vi "Update Analysis Graph.vi"(8 "error in (no error)":errorcluster, 9 "Image Series":u16[][][](array[numeric]), 10 "Analysis Image":dbl[][](array[numeric]), 11 "Analysis Graph in":refnum<class "Analysis Graph.lvclass">) -> (0 "error out":errorcluster, 1 "Image Series  out":u16[][][](array[numeric]), 2 "Cursor.Cursor Position":T1, 3 "Analysis Graph out":refnum<class "Analysis Graph.lvclass">)   [LabVIEW 2023, in "Analysis Graph.lvclass"]
uses:
  Analysis Graph.lvclass
  Analysis Graph.lvclass/Analysis Graph.ctl
  Detail Graph/Detail Graph.lvclass
  Series Graph/Series Graph.lvclass
  <vilib>/Utility/miscctls.llb/LVPointDoubleTypeDef.ctl
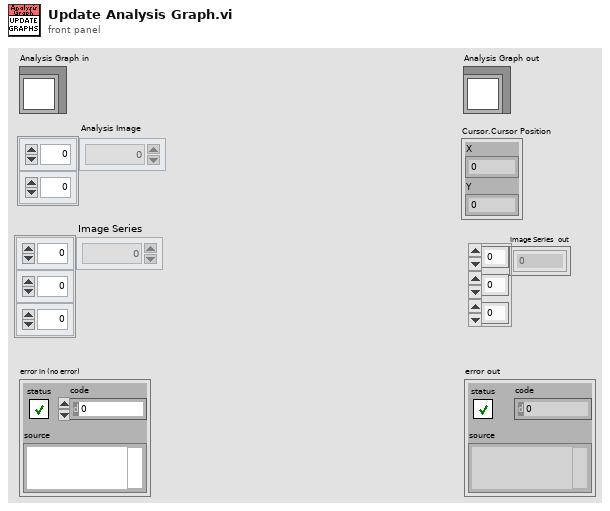
[diagram p1: front panel]
types:
  T1 = typedef "LVPointDoubleTypeDef.ctl" = cluster{"X":dbl, "Y":dbl}
  T2 = cluster{"ROI X":cluster{"Index":u32, "Length":u32}, "ROI Y":cluster{"Index":u32, "Length":u32}, "ROI Z":cluster{"Index":u32, "Length":u32}}
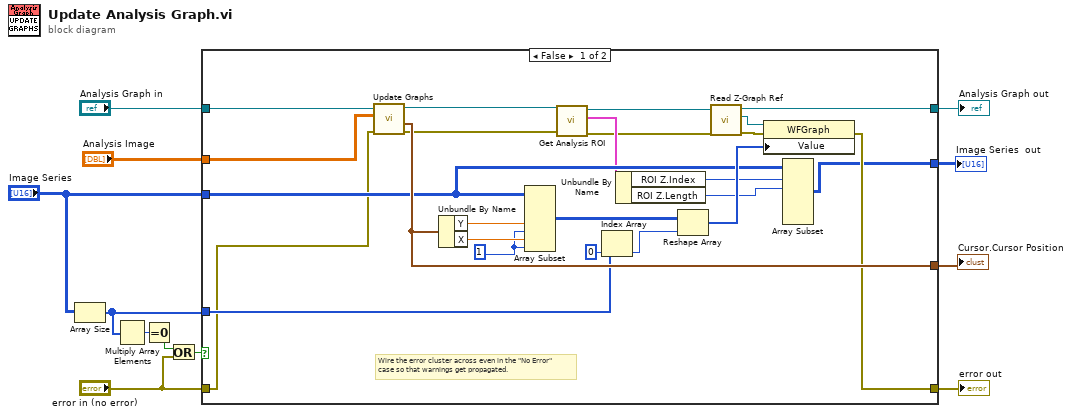
[diagram p0: block diagram]
diagram:
  n1 = Array Size(array="Image Series") -> (size(s)=w5:i32[])
  n2 = Multiply Array Elements(1:w5) -> (0:w9:i32)
  n3 = Equal To 0?(x=w9) -> (x = 0?=w8:bool)
  n4 = Or(x=w8, y="error in (no error)") -> (x .or. y?=w7:bool)
  n5 = case shown="False" w7 {
    tunnel: [w28 w39] -> w12
    tunnel: [w33 w40] -> w10
    tunnel: "Analysis Graph in" -> [w18 w40]
    tunnel: "error in (no error)" -> [w17 w39]
    tunnel: w5 -> [w23 _]
    tunnel: "Analysis Image" -> [w30 _]
    tunnel: "Image Series" -> [w26 w38]
    tunnel: [w29 _] -> w2
    tunnel: [w27 w38] -> w1
    frame False {
      w35 = 1 ("length")
      # "Wire the error cluster across even in the \"No Error\"\ncase so that warnings get propagated."
      n6 = call "Update Graphs.vi"("error in (no error)"=w17, "image"=w30, "Detail Graph in"=w18) -> ("error out"=w20:errorcluster, "Cursor.Cursor Position"=w29:T1, "Detail Graph out"=w14:refnum<class "Analysis Graph.lvclass">)  [unwired: 6 in]
      n7 = Unbundle By Name(w29) -> ("Y"=w37:dbl, "X"=w36:dbl)
      n8 = Array Subset(array=w26, index (dim 1)=w37, length (dim 1)=w35, index (dim 2)=w36, length (dim 2)=w35) -> (w22:u16[][][])  [unwired: 2 in]
      n9 = call "Get Analysis ROI.vi"("error in (no error)"=w20, "Analysis Graph in"=w14) -> ("error out"=w19:errorcluster, "ROI XYZ"=w21:T2, "Analysis Graph out"=w13:refnum<class "Analysis Graph.lvclass">)  [unwired: 7 in]
      n10 = Index Array(array=w23, index=0) -> (element=w25:i32)
      n11 = Unbundle By Name(w21) -> ("ROI Z.Index"=w16:u32, "ROI Z.Length"=w15:u32)
      n12 = Reshape Array(w22, w25) -> (w34:u16[])
      n13 = call "Read Z-Graph Ref.vi"("error in (no error)"=w19, "Series Graph in"=w13) -> ("error out"=w31:errorcluster, "Z-Graph Ref"=w32:refnum<vi>, "Series Graph out"=w33:refnum<class "Analysis Graph.lvclass">)  [unwired: 7 in]
      n14 = property class="WFGraph"(reference=w32, error in=w31, "Value"=w34) -> (error out=w28:errorcluster)  [unwired: 1 out]
      n15 = Array Subset(array=w26, index (dim 0)=w16, length (dim 0)=w15) -> (w27:u16[][][])  [unwired: 4 in]
    }
    frame True {
    }
  }
  "error out" <- w12
  "Analysis Graph out" <- w10
  "Cursor.Cursor Position" <- w2
  "Image Series  out" <- w1
